vi "LogFilter - Periodic Log Check.vi"(6 "Level (Normal)":T1, 8 "Matched Previous?":bool, 10 "Cross CSM Data In":T2, 11 "GlobalLogFilter In":refnum<class "LogFilter.lvclass">) -> (0 "Matched? (Dup)":bool, 1 "Additional Info":string[](array[string]), 2 "Cross CSM Data Out":T2, 3 "GlobalLogFilter.lvclass (Dup)":refnum<class "LogFilter.lvclass">, 4 "Filtered Status":string[](array[string]))   [LabVIEW 2017, in "Communicable State Machine.lvlib" / "LogFilter.lvclass"]
uses:
  LogFilter.lvclass
  Typedef/_CSM_GlobalLog_MSG.ctl
  Typedef/_CSM_Response Source Message.ctl
  Typedef/_CSM_GlobalLog_MSG_TYPE.ctl
  Utility/_support/Periodic String Filter Level.ctl
  LogFilter.lvclass/LogFilter.ctl
  Communicable State Machine.lvlib
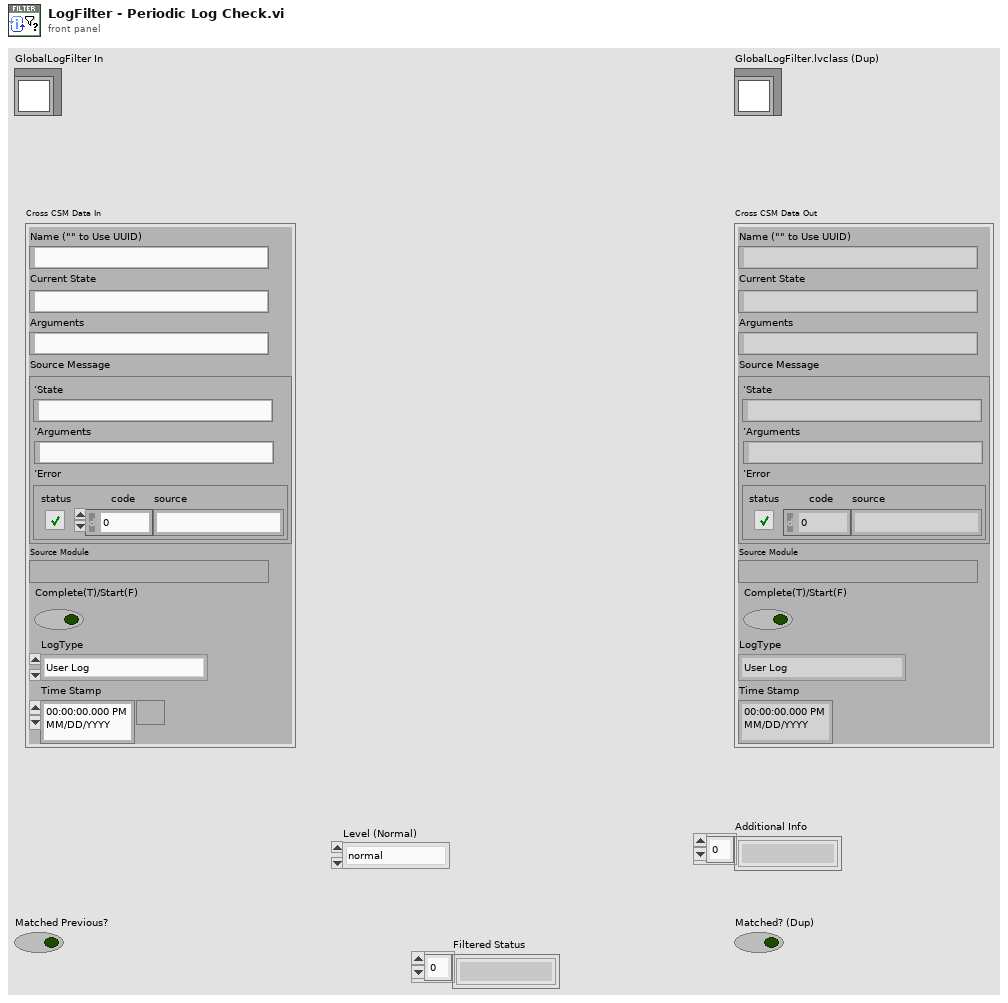
[diagram p1: front panel]
types:
  T1 = typedef "Communicable State Machine.lvlib/Periodic String Filter Level.ctl" = enum16{"normal", "L1", "L2", "L3", "L4"}
  T2 = typedef "Communicable State Machine.lvlib/_CSM_GlobalLog_MSG.ctl" = cluster{"Name (\"\" to Use UUID)":string, "Current State":string, "Arguments":string, "Source Message":T3, "Source Module":string, "Complete(T)/Start(F)":bool, "LogType":T4, "Time Stamp":timestamp}
  T3 = typedef "Communicable State Machine.lvlib/_CSM_Response Source Message.ctl" = cluster{"‘State":string, "’Arguments":string, "’Error":errorcluster}
  T4 = typedef "Communicable State Machine.lvlib/_CSM_GlobalLog_MSG_TYPE.ctl" = enum16{"User Log", "State Change", "Status", "Interrupt", "Register", "Unregister", "Error Log", "Module Created", "Module Destroyed"}
  T5 = cluster{"threashold(#/s)":dbl, "Check Peroid(s)":dbl}
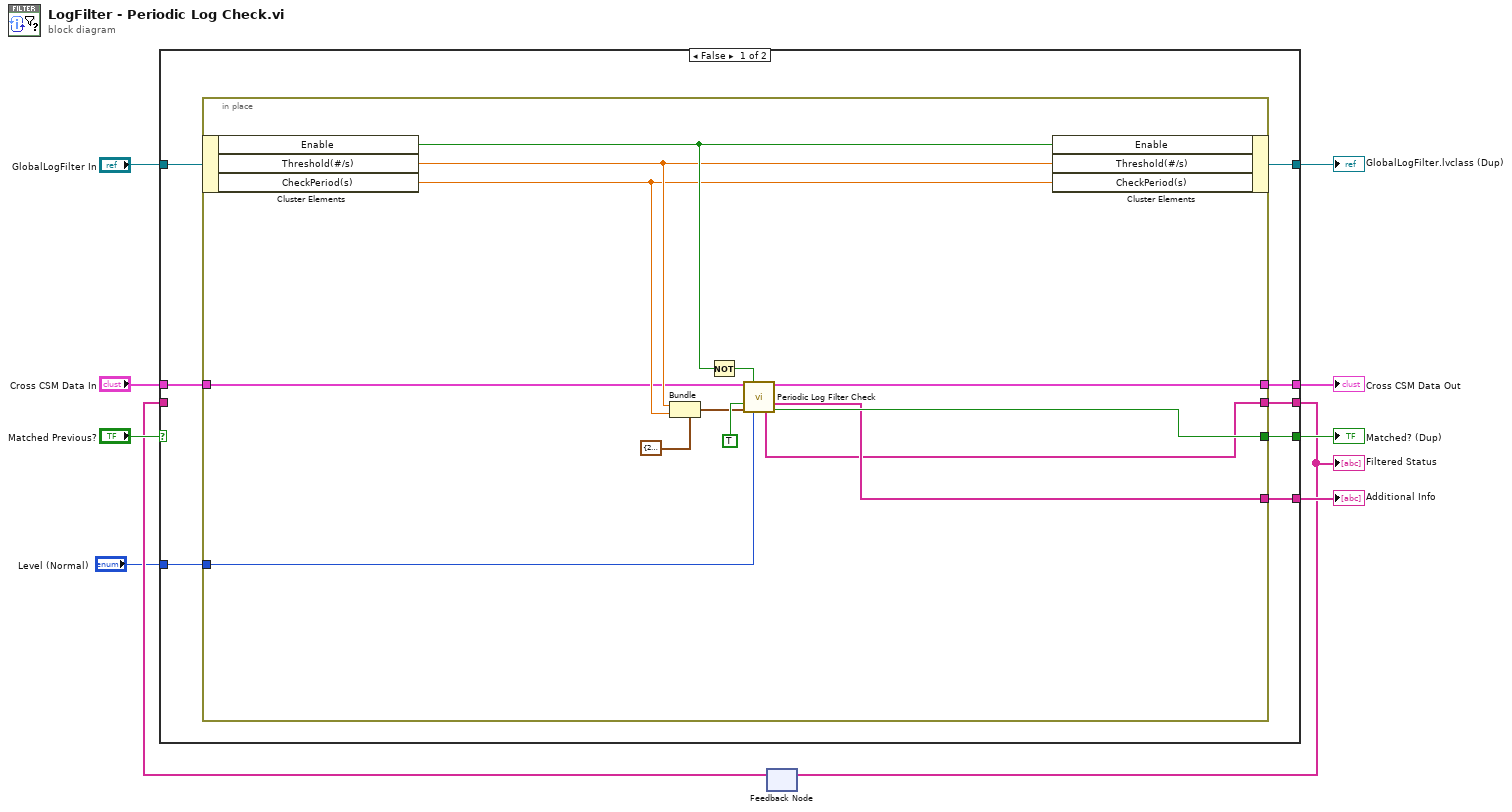
[diagram p0: block diagram]
diagram:
  n1 = feedback #1() -> (w2:string[])  [unwired: 1 in]
  n2 = case shown="False" "Matched Previous?" {
    selector: "Matched Previous?" -> [_ w35]
    tunnel: "GlobalLogFilter In" -> [w18 w33]
    tunnel: "Cross CSM Data In" -> [w17 w34]
    tunnel: [w16 w34] -> w8
    tunnel: [w15 w33] -> w7
    tunnel: [w14 w35] -> w5
    tunnel: [w13 _] -> w4
    tunnel: [w12 w32] -> w3
    tunnel: w2 -> [_ w32]
    tunnel: "Level (Normal)" -> [w11 _]
    frame False {
      n3 = in-place {
        in-place-border: w17 -> [w22]
        in-place-border: [w31] -> w16
        in-place-border: [w30] -> w14
        in-place-border: [w20] -> w13
        in-place-border: [w19] -> w12
        in-place-border: w11 -> [w21]
        n4 = in-place-cluster #2(w18) -> ("Enable"=w28:bool, "Threshold(#/s)"=w27:dbl, "CheckPeriod(s)"=w26:dbl)
        n5 = Bundle(cluster=T5 {"threashold(#/s)"=2.0, "Check Peroid(s)"=1.0} ("Settings"), "threashold(#/s)"=w27, "Check Peroid(s)"=w26) -> (w25:T5)
        n6 = Not(x=w28) -> (.not. x?=w24:bool)
        n7 = call "Periodic Log Filter Check.vi"("Cross CSM Data"=w22, "Reset?"=w24, "Remove Immediately? (F)"=TRUE ("Remove Immediately?(F)"), "Settings"=w25, "Level (Normal)"=w21) -> ("Cross CSM Data Out"=w31:T2, "Additional Info"=w20:string[], "Filtered Status"=w19:string[], "Filtered"=w30:bool)  [unwired: 6 in, 1 out]
        n8 = in-place-cluster #2("Enable"=w28, "Threshold(#/s)"=w27, "CheckPeriod(s)"=w26) -> (w15:refnum<class "LogFilter.lvclass">)
      }
    }
    frame True {
    }
  }
  "Matched? (Dup)" <- w5
  "Cross CSM Data Out" <- w8
  "GlobalLogFilter.lvclass (Dup)" <- w7
  "Additional Info" <- w4
  "Filtered Status" <- w3
  n9 = feedback-in #1(w3) -> ()
